vi "PIM Retrieve Key Array for  Config.vi"(8 "error in (no error)":errorcluster, 9 "Datasheets":T12, 10 "Key Array In":T13, 11 "Connection Refnum":T1) -> (0 "error out":errorcluster, 2 "PIM Test Parameters":T2={"Stimulus"={"C1 Pwr dBm"=0.0, "C2 Pwr dBm"=0.0, "Power Units"=enum."dBm", "Meas Type"=enum."Time", "C1 Freq MHz"=0.0, "C2 Freq MHz"=0.0, "Swept Freq Step"=0}, "Measure"={"IM Order"=0, "Direction"=0, "Averaging"=1, "ALC ON?"=TRUE, "Peak Hold?"=TRUE, "Peak last N"=1, "Ref Level dBm"=-100.0, "Ref Units"=enum."dBm", "Num Samples"=1, "Sample units"=enum."Sample(s)", "Update Rate (s)"=0.0, "DUT PORT"=enum."Port 1", "Percent (%)"=100}, "Display"={"Power Scale"={"yRange_min"=0, "yRange_max"=0}, "xRange_span"=5}} {"Stimulus"."Swept Freq Step" items=[".2", ".4", "1.0", "2.0"]; "Measure"."Averaging" items=["None", "Minimum", "Normal", "High", "Maximum"]; "Measure"."Direction" items=["Reverse", "Forward", "Auxiliary"]; "Measure"."IM Order" items=["3rd", "5th", "7th", "9th", "11th", "13th", "15th", "17th", "19th", "21st", "23rd", "25th", "27th", "29th", "31st", "33rd"]}, 3 "Connection Refnum":T1)   [LabVIEW 2011]
uses:
  ITK/utils/keyedarr.llb/Keyed Array.ctl
  Test Datasheets.ctl
  TypeDefs/PIM Test Parameters.ctl
  TypeDefs/PIM Stimulus Parameters.ctl
  BPIMCore/HW IO/PIM Sweep Step Size.ctl
  TypeDefs/PIM Measurement Parameters.ctl
  BPIMCore/HW IO/IMOrder.ctl
  BPIMCore/HW IO/MeasMode.ctl
  BPIMCore/HW IO/HW Averaging.ctl
  TypeDefs/PIM Meas Units.ctl
  BPIMCore/HW IO/DUTport.ctl
  TypeDefs/PIM Display Parameters.ctl
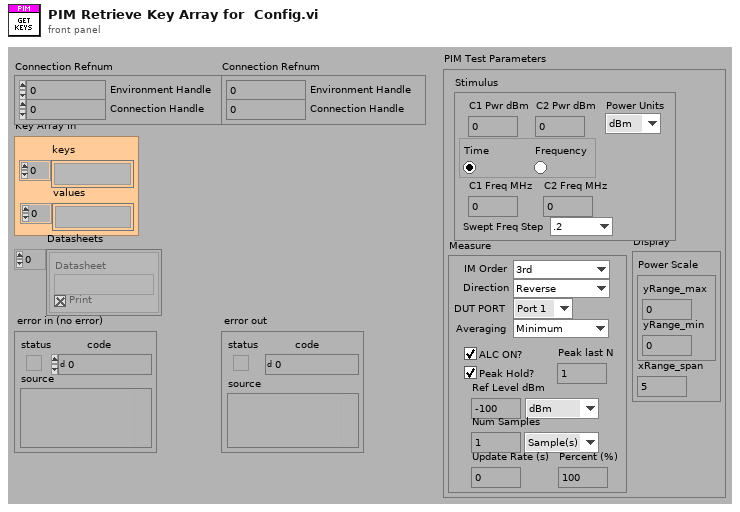
[diagram p1: front panel]
types:
  T1 = cluster{"Environment Handle":i32, "Connection Handle":i32}
  T2 = typedef "PIM Test Parameters.ctl" = cluster{"Stimulus":T3, "Measure":T5, "Display":T11}
  T3 = typedef "PIM Stimulus Parameters.ctl" = cluster{"C1 Pwr dBm":dbl, "C2 Pwr dBm":dbl, "Power Units":enum16{"dBm", "Watts"}, "Meas Type":enum32{"Time", "Frequency"}, "C1 Freq MHz":dbl, "C2 Freq MHz":dbl, "Swept Freq Step":T4}
  T4 = typedef "PIM Sweep Step Size.ctl" = u16
  T5 = typedef "PIM Measurement Parameters.ctl" = cluster{"IM Order":T6, "Direction":T7, "Averaging":T8, "ALC ON?":bool, "Peak Hold?":bool, "Peak last N":u32, "Ref Level dBm":dbl, "Ref Units":enum16{"dBm", "dBc"}, "Num Samples":u32, "Sample units":T9, "Update Rate (s)":dbl, "DUT PORT":T10, "Percent (%)":u8}
  T6 = typedef "IMOrder.ctl" = u8
  T7 = typedef "MeasMode.ctl" = u16
  T8 = typedef "HW Averaging.ctl" = u16
  T9 = typedef "PIM Meas Units.ctl" = enum16{"Sample(s)", "Second(s)", "Sweep(s)"}
  T10 = typedef "DUTport.ctl" = enum16{"Port 1", "Port 2"}
  T11 = typedef "PIM Display Parameters.ctl" = cluster{"Power Scale":cluster{"yRange_min":i32, "yRange_max":i32}, "xRange_span":u32}
  T12 = typedef "Test Datasheets.ctl" = cluster{"Datasheet":string, "Print":bool}[]
  T13 = typedef "Keyed Array.ctl" = cluster{"keys":string[], "values":string[]}
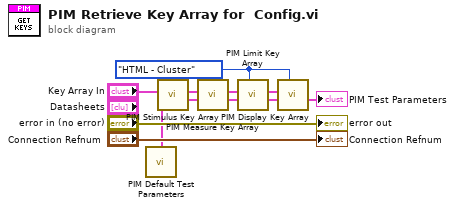
[diagram p0: block diagram]
diagram:
  w7 = enum16{"Cluster - HTML", "HTML - Cluster"}."HTML - Cluster" ("Conversion")
  n1 = call "PIM Default Test Parameters.vi"() -> ("Default PIM Test Parameters"=w3:T2)
  n2 = call "PIM Stimulus Key Array.vi"("Conversion"=w7, "PIM Test Parameters"=w3, "Key Array In"="Key Array In") -> ("PIM Test Parameters (out)"=w4:T2, "Key Array Out"=w10:T13)  [unwired: 4 in]
  n3 = call "PIM Measure Key Array.vi"("Conversion"=w7, "PIM Test Parameters"=w4, "Key Array In"=w10) -> ("PIM Test Parameters (out)"=w5:T2, "Key Array Out"=w9:T13)  [unwired: 4 in]
  n4 = call "PIM Limit Key Array.vi"("Conversion"=w7, "PIM Test Parameters"=w5, "Key Array In"=w9) -> ("PIM Test Parameters (out)"=w6:T2, "Key Array Out"=w8:T13)  [unwired: 4 in]
  n5 = call "PIM Display Key Array.vi"("Conversion"=w7, "PIM Test Parameters"=w6, "Key Array In"=w8) -> ("PIM Test Parameters (out)"=→"PIM Test Parameters":T2)  [unwired: 4 in, 1 out]
  "error out" <- "error in (no error)"
  "Connection Refnum" <- "Connection Refnum"
